vi "OR_deadZone.vi"(10 "x in":dbl, 11 "Reset 0 Pos":bool) -> (3 "x out":dbl)   [LabVIEW 2014]
panel:
  in  "DeadZoneAmplitude":dbl=5.0
  in  "Zero Angle":dbl
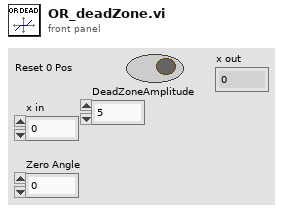
[diagram p1: front panel]
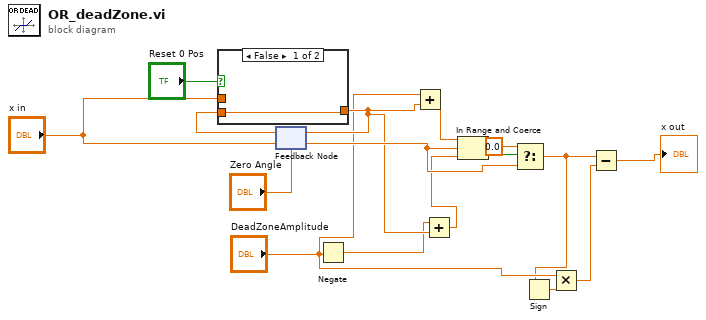
[diagram p0: block diagram]
diagram:
  n1 = feedback #1("Zero Angle") -> (w14:dbl)
  n2 = case shown="False" "Reset 0 Pos" {
    tunnel: [w16 w17] -> w7
    tunnel: "x in" -> [_ w17]
    tunnel: w14 -> [w16 _]
    frame False {
    }
    frame True {
    }
  }
  n3 = feedback-in #1(w7) -> ()
  n4 = Negate(x="DeadZoneAmplitude") -> (-x=w6:dbl)
  n5 = Add(x="DeadZoneAmplitude", y=w7) -> (x+y=w10:dbl)
  n6 = Add(x=w6, y=w7) -> (x+y=w11:dbl)
  n7 = In Range and Coerce(upper limit=w10, x="x in", lower limit=w11) -> (In Range?=w8:bool)  [unwired: 1 out]
  n8 = Select(t=0.0, s=w8, f="x in") -> (s? t:f=w2:dbl)
  n9 = Sign(1:w2) -> (0:w3:dbl)
  n10 = Multiply(x="DeadZoneAmplitude", y=w3) -> (x*y=w4:dbl)
  n11 = Subtract(x=w2, y=w4) -> (x-y=→"x out":dbl)
